vi "SaveConfig.vi"(10 "ControlsToSave":refnum<vi>[](array[refnum]), 11 "Path":path) -> ()   [LabVIEW 2015]
uses:
  <vilib>/Utility/config.llb/NI_LVConfig.lvlib
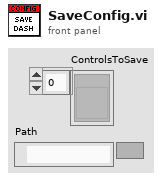
[diagram p1: front panel]
types:
  T1 = typedef "NI_LVConfig.lvlib/Config Data RefNum.ctl" = refnum<k1>
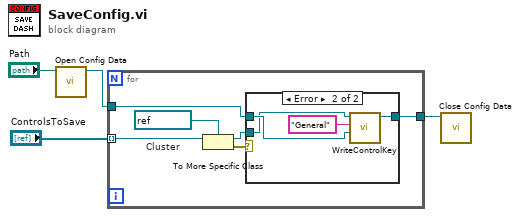
[diagram p0: block diagram]
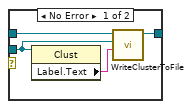
[diagram p2: hidden frame]
diagram:
  n1 = call <vilib>:"Open Config Data.vi"("configuration file path"="Path") -> ("refnum"=w2:T1)  [unwired: 8 in, 2 out]
  n2 = for {
    tunnel: "ControlsToSave" -> [w10] mode=indexing
    tunnel: w2 -> [w7]
    tunnel: [w5] -> w1
    w9 = refnum<vi> refnum  # Cluster
    n3 = To More Specific Class(target class=w9, reference=w10) -> (specific class reference=w6:refnum<vi>, error out=w8:errorcluster)  [unwired: 1 in]
    n4 = case shown="Error" w8 {
      tunnel: w7 -> [w14 w18]
      tunnel: w6 -> [w13 w17]
      tunnel: [w11 w15] -> w5
      frame No Error {
        n5 = property class="Clust"(reference=w13) -> ("Label.Text"=w12:string)  [unwired: 1 in, 2 out]
        n6 = call "WriteClusterToFile.vi"("Name"=w12, "Cluster in"=w13, "ConfigIn"=w14) -> ("ConfigOut"=w11:T1)  [unwired: 8 in]
      }
      frame Error {
        n7 = call "WriteControlKey.vi"("ConfigFile"=w18, "section"="General", "Control in"=w17) -> ("ConfigFile out"=w15:T1)  [unwired: 8 in]
      }
    }
  }
  n8 = call <vilib>:"Close Config Data.vi"("refnum"=w1) -> ()  [unwired: 9 in, 2 out]
